vi "Update Status.vi"(8 "error in (no error)":errorcluster caption="entrée d'erreur (pas d'erreur)", 10 "DAQmx Tasks":T1(array[cluster]), 11 "DAQmxTaskContainer en entrée":refnum<class "DAQmxTaskContainer.lvclass">) -> (0 "error out":errorcluster caption="sortie d'erreur", 2 "DAQmx Tasks out":T1(array[cluster]), 3 "DAQmxTaskContainer en sortie":refnum<class "DAQmxTaskContainer.lvclass">)   [LabVIEW 2015, in "DAQmxTaskContainer.lvclass"]
uses:
  DAQmxTaskContainer.lvclass
  DAQmxTaskContainer.lvclass/DAQmxTaskContainer.ctl
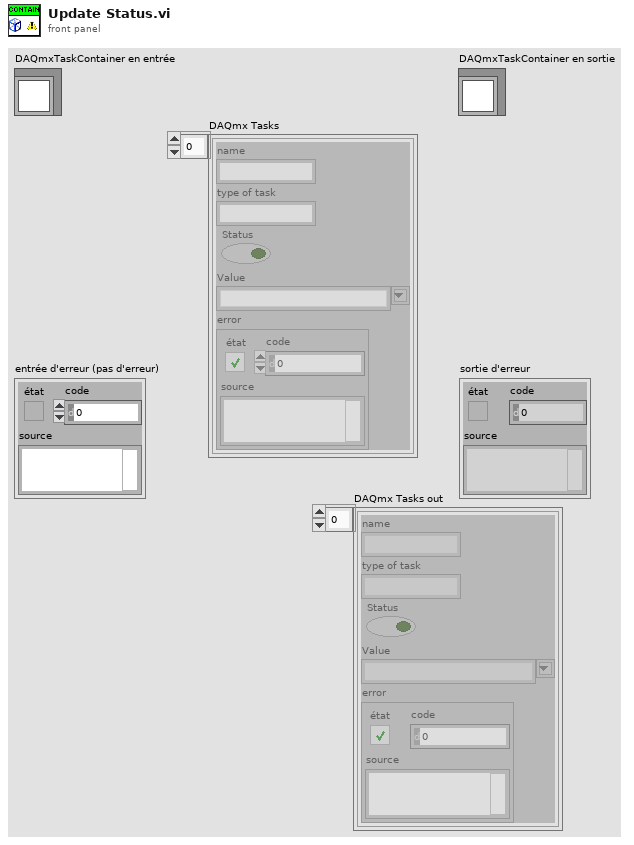
[diagram p1: front panel]
types:
  T1 = cluster{"name":string, "type of task":string, "Status":bool, "Value":string, "error":errorcluster}[]
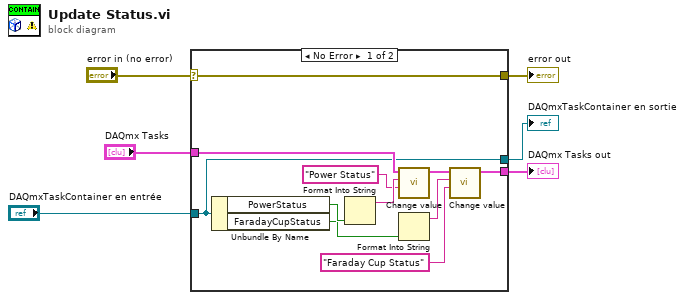
[diagram p0: block diagram]
diagram:
  n1 = case shown="No Error" "error in (no error)" {
    selector: "error in (no error)" -> [w17 w20]
    tunnel: [w17 w20] -> w5
    tunnel: [w15 w19] -> w3
    tunnel: "DAQmxTaskContainer en entrée" -> [w15 w19]
    tunnel: "DAQmx Tasks" -> [w16 w18]
    tunnel: [w7 w18] -> w1
    frame No Error {
      n2 = Unbundle By Name(w15) -> ("PowerStatus"=w14:bool, "FaradayCupStatus"=w13:bool)
      n3 = Format Into String(w14) -> (resulting string=w12:string)  [unwired: 3 in, 1 out]
      n4 = call "Change value.vi"("Task name"="Power Status", "Data string"=w12, "DAQmx Tasks"=w16) -> ("tableau en sortie"=w9:T1)  [unwired: 8 in]
      n5 = Format Into String(w13) -> (resulting string=w10:string)  [unwired: 3 in, 1 out]
      n6 = call "Change value.vi"("Task name"="Faraday Cup Status", "Data string"=w10, "DAQmx Tasks"=w9) -> ("tableau en sortie"=w7:T1)  [unwired: 8 in]
    }
    frame Error {
    }
  }
  "error out" <- w5
  "DAQmxTaskContainer en sortie" <- w3
  "DAQmx Tasks out" <- w1
